vi "ARydh_get_voltage -- V1.vi"(4 "Oscillator (0)":u16, 8 "Error In":errorcluster, 9 "timeconstant (s)":dbl=0.006, 10 "Freq IN (Hz)":dbl=40000.0 format="%#_13g", 11 "MCL object IN":T1) -> (0 "Error Out":errorcluster, 1 "z out (V)":cdb, 2 "Freq out (Hz)":dbl=40000.0 format="%#_13g", 3 "MCL object OUT":T1)   [LabVIEW 2021]
uses:
  nanocal/Nanocalorimetry/data/MCL.lvlibp/SynkTek FPGA/FPGA_SharedResources/FPGASharedResources_Lockin_Typedef.ctl
  Arydh  lockin fields.ctl
  nanocal/Nanocalorimetry/data/MCL.lvlibp/SynkTek FPGA/FPGA_SharedResources/FPGASharedResources_FreqCtrl_FreqGenTypedef.ctl
  nanocal/Nanocalorimetry/data/MCL.lvlibp/SynkTek FPGA/FPGA_SharedResources/FPGASharedResources_PhaseShiftCtrl_Typedef.ctl
  nanocal/Nanocalorimetry/data/MCL.lvlibp/SynkTek Host/LIdata/LIData_DataReadings_typedef.ctl
  nanocal/Nanocalorimetry/data/MCL.lvlibp/MCL library/MCL_DataRef.ctl
panel:
  out "Phase OUT (deg)":dbl=40000.0 format="%#_13g"
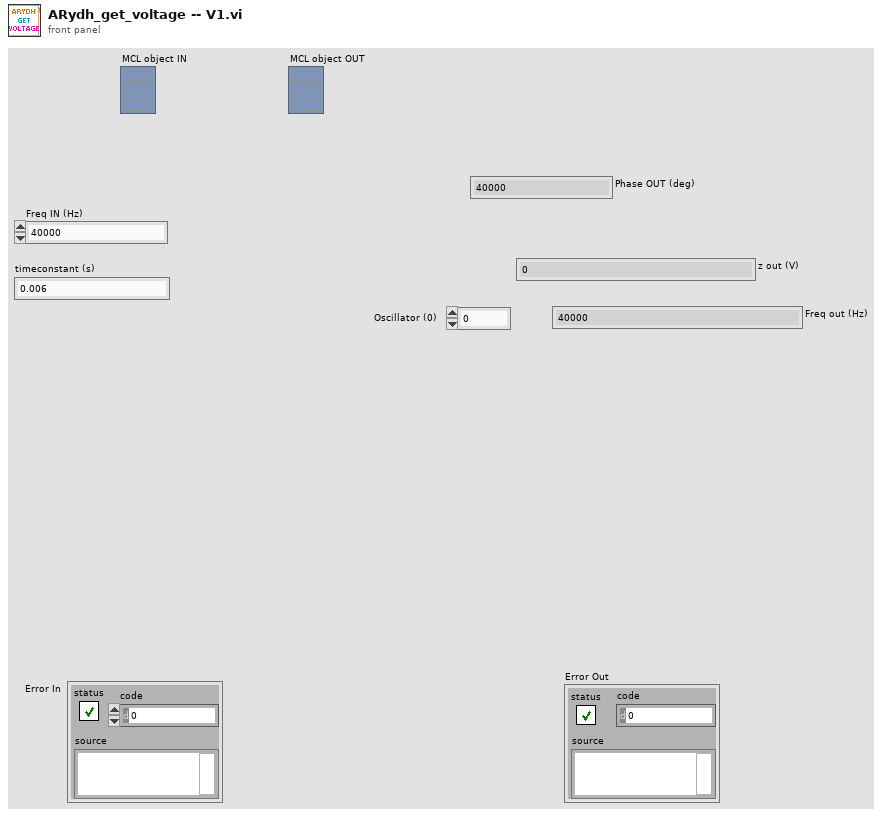
[diagram p1: front panel]
types:
  T1 = typedef "MCL.lvlibp/MCL_DataRef.ctl" = refnum<vi>
  T2 = typedef "Arydh  lockin fields.ctl" = enum16{"AV1", "AV2", "BV1", "BV2", "CV1", "CV2", "DV1", "DV2", "EV1", "EV2", "AI", "BI", "CI", "DI", "EI", "int"}
  T3 = typedef "MCL.lvlibp/FPGA_SharedResources.lvlib/FPGASharedResources_Lockin_Typedef.ctl" = enum8{"Lock-in set L1", "Lock-in set L2"}
  T4 = typedef "MCL.lvlibp/FPGA_SharedResources.lvlib/FPGASharedResources_PhaseShiftCtrl_Typedef.ctl" = enum8{"Phase 1", "Phase 2", "Phase 3", "Phase 4", "Phase 5", "Phase 6", "Phase 7", "Disabled"}
  T5 = typedef "MCL.lvlibp/FPGA_SharedResources.lvlib/FPGASharedResources_FreqCtrl_FreqGenTypedef.ctl" = enum8{"Frequency 1", "Frequency 2", "Frequency 3", "Frequency 4", "Frequency 5", "Frequency 6: PLL 1", "Frequency 7: PLL 2", "Frequency 8"}
  T6 = typedef "MCL.lvlibp/LIData.lvlib/LIData_DataReadings_typedef.ctl" = cluster{"DC":dbl[], "X":dbl[], "Y":dbl[], "R":dbl[], "theta (deg)":dbl[]}
  T7 = typedef "MCL.lvlibp/LIData.lvlib/LIData_Readings_Typedef.ctl" = cluster{"dt (s)":dbl, "Cycles per sample":dbl, "Sync index":dbl, "Point number":dbl, "Lock-in f (Hz)":dbl, "Module data":cluster{"Digital in f (Hz)":dbl, "Digital out f (Hz)":dbl, "Amplitude (Vrms)":dbl, "Output offset (V)":dbl}[], "PLL 1 (Hz)":dbl, "PLL 2 (Hz)":dbl, "Composite 1 (Hz)":dbl}
  T8 = cluster{"Digital in f (Hz)":dbl, "Digital out f (Hz)":dbl, "Amplitude (Vrms)":dbl, "Output offset (V)":dbl}[]
  T9 = cluster{"Digital in f (Hz)":dbl, "Digital out f (Hz)":dbl, "Amplitude (Vrms)":dbl, "Output offset (V)":dbl}
  T10 = typedef "MCL.lvlibp/LIControl.lvlib/LIControl_PhaseShiftCtrl_typedef.ctl" = dbl
  T11 = typedef "MCL.lvlibp/LIControl.lvlib/LIControl_FreqCtrl_typedef.ctl" = cluster{"Frequency (Hz)":dbl, "Ramp changes":bool, "Ramp time const. (s)":T12}
  T12 = typedef "MCL.lvlibp/LIControl.lvlib/LIControl_LockinTimeConstant_typedef.ctl" = dbl
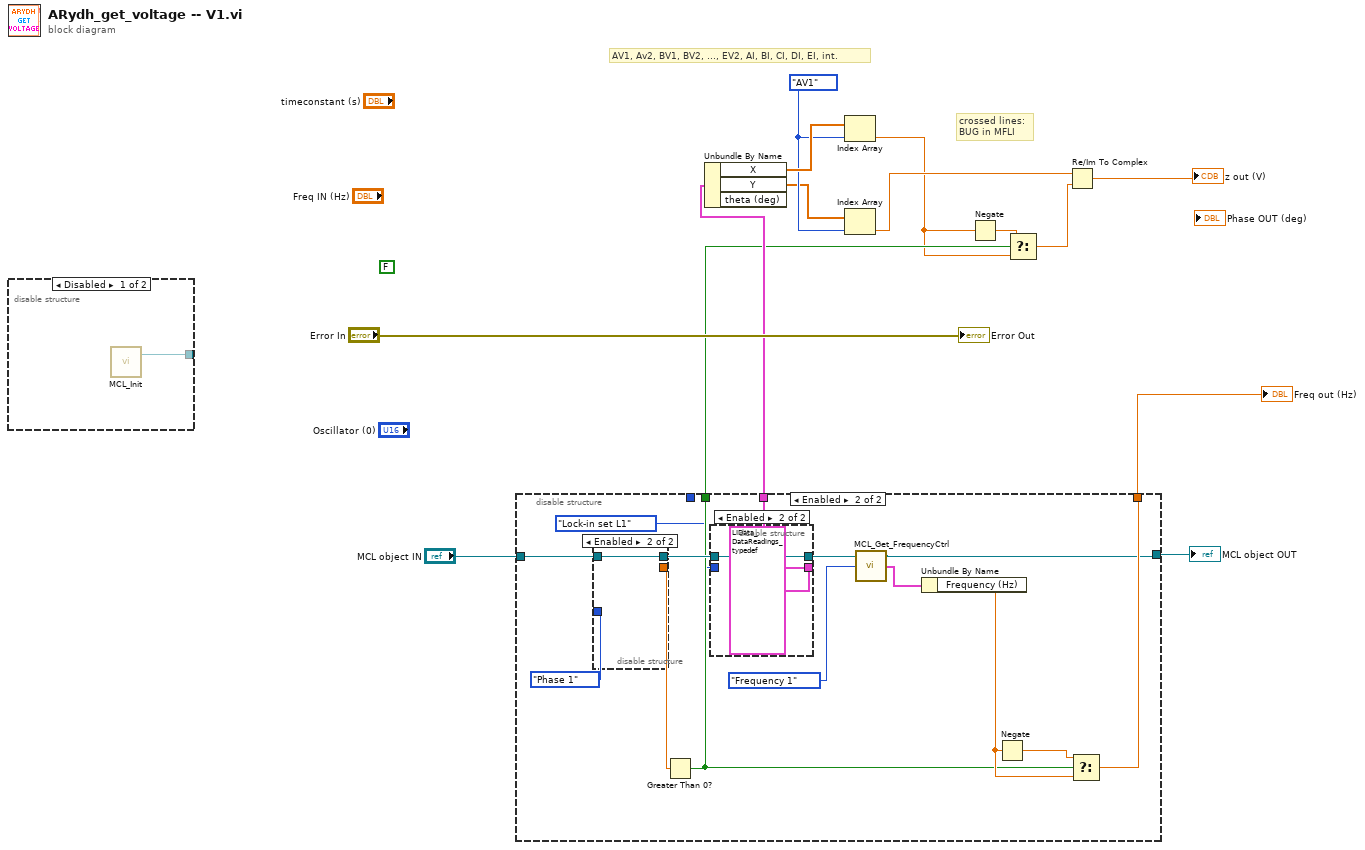
[diagram p0: block diagram]
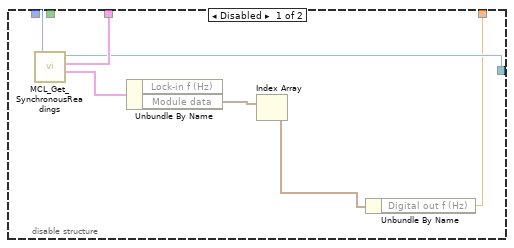
[diagram p3: hidden frame]
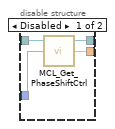
[diagram p4: hidden frame]
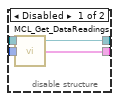
[diagram p5: hidden frame]
diagram:
  w12 = Arydh__lockin_fields."AV1"
  (unwired) FALSE
  # "AV1, Av2, BV1, BV2, ..., EV2, AI, BI, CI, DI, EI, int."
  # "crossed lines:\nBUG in MFLI"
  n1 = disable-structure shown="Disabled" {
    disable-tunnel: [w15 _] -> _
    frame Disabled {
      n2 = call "MCL_Init.vi"() -> ("MCL object"=w15:T1)  [unwired: 2 in, 1 out]
    }
    frame Enabled {
    }
  }
  n3 = disable-structure shown="Enabled" {
    disable-tunnel: [w23 w37] -> w9
    disable-tunnel: [w18 w25] -> w1
    disable-tunnel: [w17 w30] -> w8
    disable-tunnel: _ -> [w16 _]
    disable-tunnel: "MCL object IN" -> [_ w36]
    disable-tunnel: [_ w29] -> w7
    frame Disabled {
      n4 = call "MCL_Get_SynchronousReadings.vi"("Lockin"=w16) -> (0:"MCL object"=w19:T1, 3:"MCL object"=w18:T1, "DataReadings"=w23:T6, "GeneralReadings"=w22:T7)  [unwired: 1 in, 1 out]
      n5 = Unbundle By Name(w22) -> ("Module data"=w21:T8)  [unwired: 1 out]
      n6 = Index Array(array=w21) -> (element=w20:T9)  [unwired: 1 in]
      n7 = Unbundle By Name(w20) -> ("Digital out f (Hz)"=w17:dbl)
    }
    frame Enabled {
      n8 = disable-structure shown="Enabled" {
        disable-tunnel: w36 -> [w41 w42]
        disable-tunnel: [w40 w42] -> w35
        disable-tunnel: FPGASharedResources_PhaseShiftCtrl_Typedef."Phase 1" ("PhaseShift") -> [w39 _]
        disable-tunnel: [w38 _] -> w33
        frame Disabled {
          n9 = call "MCL_Get_PhaseShiftCtrl.vi"("PhaseShift"=w39, "MCL object"=w41) -> ("Phase shift (deg)"=w38:T10, "MCL object"=w40:T1)  [unwired: 1 in, 1 out]
        }
        frame Enabled {
        }
      }
      n10 = Greater Than 0?(x=w33) -> (x > 0?=w29:bool)
      n11 = disable-structure shown="Enabled" {
        disable-tunnel: [w46 T6 {"DC"=[0.0, 0.0, 0.0, 0.0, 0.0, 0.0, 0.0, 0.0, 0.0, 0.0, 0.0, 0.0, 0.0, 0.0, 0.0, 0.0], "X"=[0.0, 0.0, 0.0, 0.0, 0.0, 0.0, 0.0, 0.0, 0.0, 0.0, 0.0, 0.0, 0.0, 0.0, 0.0, 0.0], "Y"=[0.0, 0.0, 0.0, 0.0, 0.0, 0.0, 0.0, 0.0, 0.0, 0.0, 0.0, 0.0, 0.0, 0.0, 0.0, 0.0], "R"=[0.0, 0.0, 0.0, 0.0, 0.0, 0.0, 0.0, 0.0, 0.0, 0.0, 0.0, 0.0, 0.0, 0.0, 0.0, 0.0], "theta (deg)"=[0.0, 0.0, 0.0, 0.0, 0.0, 0.0, 0.0, 0.0, 0.0, 0.0, 0.0, 0.0, 0.0, 0.0, 0.0, 0.0]} ("DataReadings")] -> w37
        disable-tunnel: [w45 w47] -> w27
        disable-tunnel: w35 -> [w44 w47]
        disable-tunnel: FPGASharedResources_Lockin_Typedef."Lock-in set L1" ("Lockin") -> [w43 _]
        frame Disabled {
          n12 = call "MCL_Get_DataReadings.vi"("Lockin"=w43, "MCL object"=w44) -> ("DataReadings"=w46:T6, "MCL object"=w45:T1)  [unwired: 1 in, 1 out]
        }
        frame Enabled {
        }
      }
      n13 = call "MCL_Get_FrequencyCtrl.vi"("Frequency generator"=FPGASharedResources_FreqCtrl_FreqGenTypedef."Frequency 1", "MCL object"=w27) -> ("FrequencyCtrl"=w24:T11, "MCL object"=w25:T1)  [unwired: 1 in, 1 out]
      n14 = Unbundle By Name(w24) -> ("Frequency (Hz)"=w31:dbl)
      n15 = Negate(x=w31) -> (-x=w32:dbl)
      n16 = Select(t=w32, s=w29, f=w31) -> (s? t:f=w30:dbl)
    }
  }
  "Freq out (Hz)" <- w8
  "MCL object OUT" <- w1
  n17 = Unbundle By Name(w9) -> ("X"=w13:dbl[], "Y"=w11:dbl[])  [unwired: 1 out]
  n18 = Index Array(array=w13, index=w12) -> (element=w4:dbl)
  n19 = Index Array(array=w11, index=w12) -> (element=w5:dbl)
  n20 = Negate(x=w4) -> (-x=w6:dbl)
  n21 = Select(t=w6, s=w7, f=w4) -> (s? t:f=w3:dbl)
  n22 = Re/Im To Complex(1:w3, 2:w5) -> (0:→"z out (V)":cdb)
  "Error Out" <- "Error In"
